vi "Get settings chain.vi"(8 "error in (no error)":errorcluster, 11 "ExampleClassCBase in":refnum<class "ExampleClassC.lvclass">) -> (0 "error out":errorcluster, 1 "class name":string[](array[string]), 2 "settings":variant[](array[variant]), 3 "ExampleClassCBase out":refnum<class "ExampleClassC.lvclass">)   [LabVIEW 2012, in "ExampleClassC.lvclass"]
doc: "Returns an array of variants containing the settings clusters of each class in the inheritance chain (lowest child class first), together with an array of all class names in the inheritance chain.\n\nFor classes without settings cluster, the settings chain contains empty variants."
uses:
  ExampleClassC.lvclass
  <vilib>/Distrio/Murmex/Murmex/Murmex.lvclass
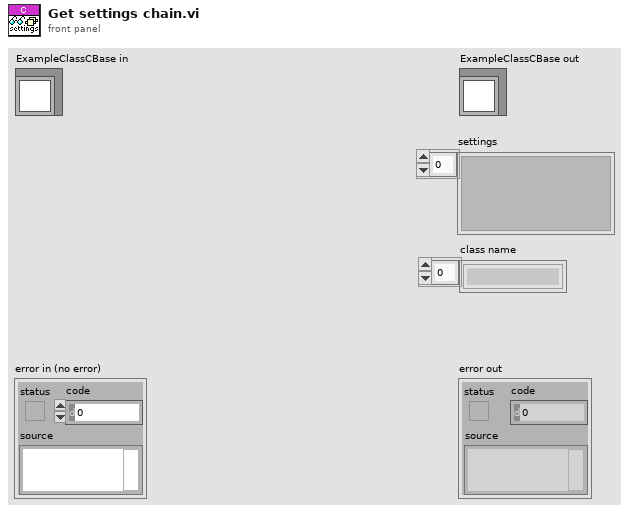
[diagram p1: front panel]
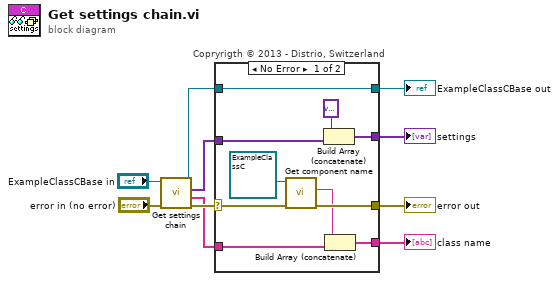
[diagram p0: block diagram]
diagram:
  n1 = call-parent "Get settings chain.vi"("error in (no error)"="error in (no error)", "MurmexBase in"="ExampleClassCBase in") -> ("error out"=w8:errorcluster, "class name"=w2:string[], "settings"=w6:variant[], "MurmexBase out"=w7:refnum<class "ExampleClassC.lvclass">)  [unwired: 6 in]
  n2 = case "Copryrigth © 2013 - Distrio, Switzerland" shown="No Error" w8 {
    selector: w8 -> [w20 w22]
    tunnel: [w19 w22] -> w1
    tunnel: [w12 w21] -> w5
    tunnel: w7 -> [w12 w21]
    tunnel: [w17 _] -> w3
    tunnel: [w16 _] -> w4
    tunnel: w6 -> [w14 _]
    tunnel: w2 -> [w13 _]
    frame No Error {
      n3 = call <vilib>:"Get component name.vi"("error in (no error)"=w20, "Murmex in"=refnum<class "ExampleClassC.lvclass"> refnum ("ExampleClassCBase in")) -> ("error out"=w19:errorcluster, "component name"=w18:string)  [unwired: 7 in, 1 out]
      n4 = Build Array (concatenate)(variant ("variant"), w14) -> (w16:variant[])
      n5 = Build Array (concatenate)(w18, w13) -> (w17:string[])
    }
    frame Error {
    }
  }
  "error out" <- w1
  "ExampleClassCBase out" <- w5
  "settings" <- w4
  "class name" <- w3
